vi "GetAllPaths.vi"(0 "LocalName":string) -> (1 "Hard Path":path, 3 "User Documents":path)   [LabVIEW 2012]
doc: "Gets the paths for LVROS, the servers, _BlankServer, and the Master Console"
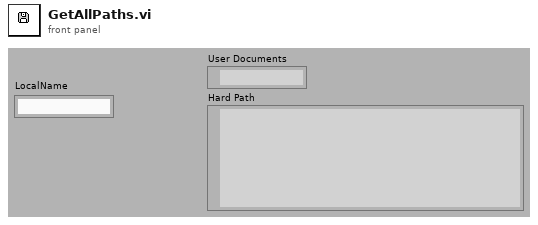
[diagram p1: front panel]
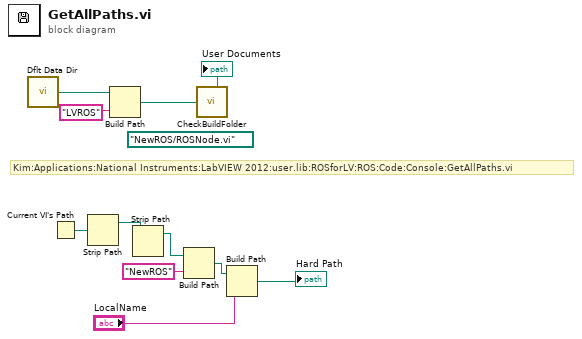
[diagram p0: block diagram]
diagram:
  (unwired) path "NewROS/ROSNode.vi"
  # "Kim:Applications:National Instruments:LabVIEW 2012:user.lib:ROSforLV:ROS:Code:Console:GetAllPaths.vi"
  n1 = call <vilib>:"Dflt Data Dir.vi"() -> ("App:Default Data Directory"=w8:path)
  n2 = Current VI's Path() -> (path=w10:path)
  n3 = Strip Path(path=w10) -> (stripped path=w6:path)  [unwired: 1 out]
  n4 = Build Path(base path=w8, name or relative path="LVROS") -> (appended path=w7:path)
  "User Documents" <- w7
  n5 = Strip Path(path=w6) -> (stripped path=w5:path)  [unwired: 1 out]
  n6 = Build Path(base path=w5, name or relative path="NewROS") -> (appended path=w4:path)
  n7 = call <userlib>:"CheckBuildFolder.vi"("appended path"=w7) -> ()  [unwired: 1 in]
  n8 = Build Path(base path=w4, name or relative path="LocalName") -> (appended path=→"Hard Path":path)
